vi "Custom gRPC Service Core.vi"(6 "Event Registration Refnum in":refnum<event-registration>, 11 "Node In":refnum<class "BLS Cycler Template.lvclass">) -> (2 "Server Stop":bool, 3 "Node out":refnum<class "BLS Cycler Template.lvclass">, 4 "Event Registration Refnum out":refnum<event-registration>)   [LabVIEW 2023, in "BLS Cycler Template.lvlib" / "BLS Cycler Template.lvclass"]
uses:
  BLS Cycler Template.lvclass
  C:/Program Files/National Instruments/LabVIEW 2023/vi.lib/ADAS Replay HIL/Template Node/Plugin/Template Node/Template Node.lvclass
  Custom gRPC/BLSCyclerTemplateService_server/RPC Service/BLSCyclerTemplateService/typeDefs/Server gRPC UEs.ctl
  <vilib>/gRPC/LabVIEW gRPC Library/Server API/typeDefs/gRPCId Cluster.ctl
  <vilib>/gRPC/LabVIEW gRPC Library/Shared/grpcId.ctl
  Custom gRPC/BLSCyclerTemplateService_server/RPC Messages/adas_Status.ctl
  <vilib>/ADAS Replay HIL/Template Node/Plugin/Template Node/Template Node.lvclass/Template Node.ctl
  <vilib>/ADAS Replay HIL/ADAS Plugin Utilities/AdasLvTemplate/AdasLvTemplate.lvclass/AdasLvTemplate.ctl
  <vilib>/ADAS Replay HIL/ADAS Plugin Utilities/AdasLvTemplate/AdasLvTemplate.lvclass
  <vilib>/ADAS Replay HIL/Template Node/Plugin/Template Node/Template Node.lvclass
  Custom gRPC/BLSCyclerTemplateService_server/BLSCyclerTemplateService_server.lvlib
  Custom gRPC/BLSCyclerTemplateService_server/RPC Service/BLSCyclerTemplateService/BLSCyclerTemplateService.lvclass
  <vilib>/gRPC/LabVIEW gRPC Library/grpc-lvsupport-release.lvlib
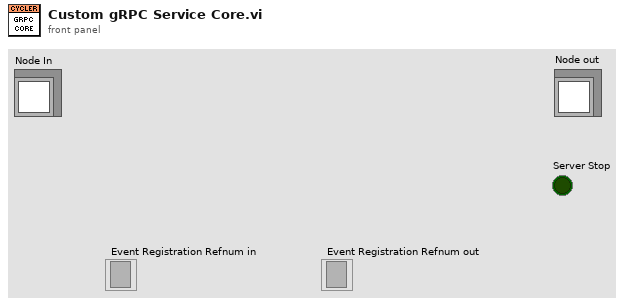
[diagram p1: front panel]
types:
  T1 = typedef "BLSCyclerTemplateService_server.lvlib/adas_Status.ctl" = cluster{"Code":i32, "Message":string}
  T2 = typedef "grpc-lvsupport-release.lvlib/grpcId.ctl" = u64
  T3 = typedef "BLSCyclerTemplateService_server.lvlib/adas_SetNumberRequest.ctl" = cluster{"SetNumber":u32}
  T4 = typedef "CIPC_buffer.lvlib/Buffer Reference.ctl" = cluster{"cipc_buffer_ref":u64, "info":T5, "settings":cluster{"prepend_array_size":bool}}
  T5 = typedef "CIPC_buffer.lvlib/Info.ctl" = cluster{"name":string, "description":string, "size":T6, "encoder":cluster{"name":string, "version":u32, "data":string}}
  T6 = typedef "CIPC_buffer.lvlib/Info Size.ctl" = cluster{"el_size_max":u32, "nr_elements":u32, "nr_elements_in_memory":u32, "frame_size":u32, "order_of_frame_size":u32, "buffer_size":u32, "order_of_buffer_size":u32}
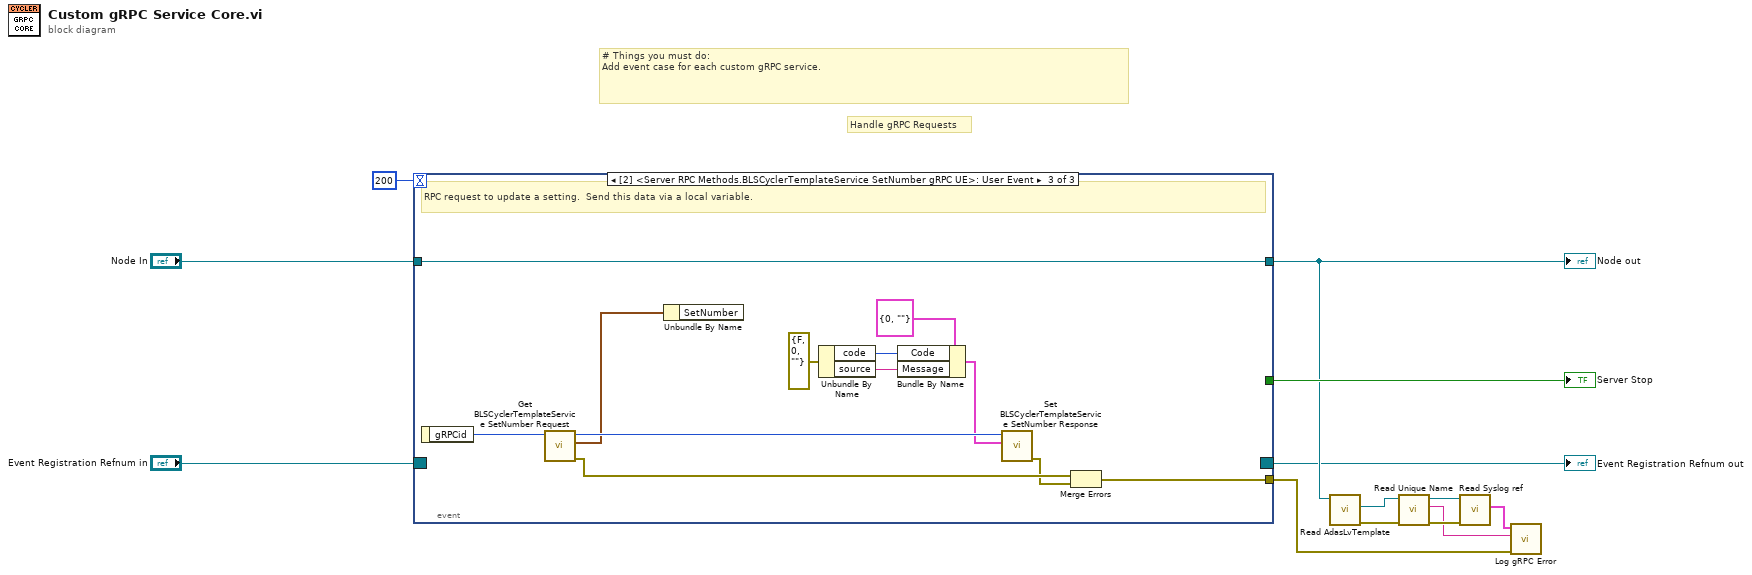
[diagram p0: block diagram]
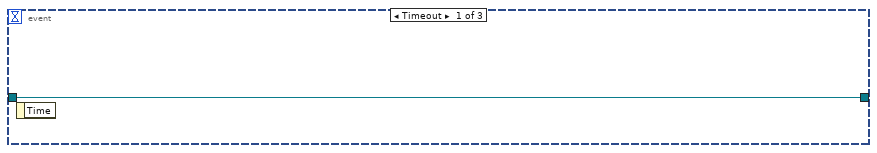
[diagram p2: hidden frame]
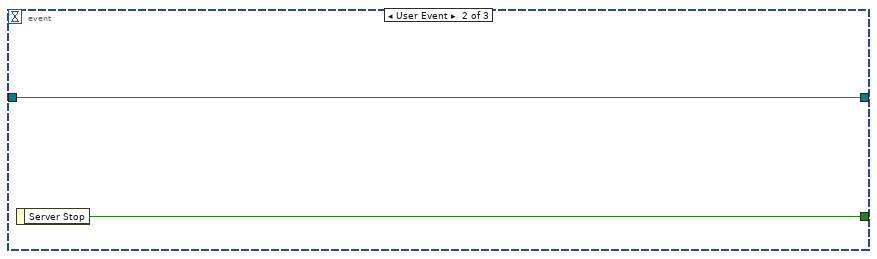
[diagram p3: hidden frame]
diagram:
  # "# Things you must do:\nAdd event case for each custom gRPC service."
  # "Handle gRPC Requests"
  n1 = event "RPC Methods Event Structure" shown="[2] <Server RPC Methods.BLSCyclerTemplateService SetNumber gRPC UE>: User Event" {
    selector: "Event Registration Refnum in" -> [_ _ _]
    dyn-events: [_ _ _] -> w1
    timeout: 200 -> [_ _ _]
    tunnel: [_ w16 _] -> w12
    tunnel: [_ _ w23] -> w4
    tunnel: "Node In" -> [w14 w15 w22]
    tunnel: [w14 w15 w22] -> w3
    event Timeout {
      n2 = event-data() -> ()  [unwired: 1 in, 1 out]
    }
    event User Event {
      n3 = event-data() -> ("Server Stop"=w16:bool)  [unwired: 1 in]
    }
    event User Event {
      # "RPC request to update a setting.  Send this data via a local variable."
      n4 = event-data() -> ("gRPCid"=w28:T2)  [unwired: 1 in]
      n5 = call "Get BLSCyclerTemplateService SetNumber Request.vi"("gRPCid in"=w28) -> ("error out"=w25:errorcluster, "Message Data"=w26:T3, "gRPCid out"=w27:T2)  [unwired: 8 in]
      n6 = Unbundle By Name(w26) -> ()  [unwired: 1 out]
      n7 = Unbundle By Name(errorcluster {"status"=FALSE, "code"=0, "source"=""} ("input cluster")) -> ("code"=w20:i32, "source"=w19:string)
      n8 = Bundle By Name(cluster=T1 {"Code"=0, "Message"=""} ("Message Data"), "Code"=w20, "Message"=w19) -> (w18:T1)
      n9 = call "Set BLSCyclerTemplateService SetNumber Response.vi"("Message Data"=w18, "gRPCid in"=w27) -> ("error out"=w24:errorcluster)  [unwired: 9 in]
      n10 = Merge Errors(w25, w24) -> (w23:errorcluster)
    }
  }
  "Server Stop" <- w12
  "Node out" <- w3
  "Event Registration Refnum out" <- w1
  n11 = call <vilib>:"Read AdasLvTemplate.vi"("Template Node in"=w3) -> ("error out"=w10:errorcluster, "AdasLvTemplate.lvlib:AdasLvTemplate.lvclass"=w11:refnum<class "AdasLvTemplate.lvclass">)  [unwired: 8 in, 1 out]
  n12 = call <vilib>:"Read Unique Name.vi"("error in"=w10, "AdasLvTemplate in"=w11) -> ("error out"=w9:errorcluster, "Unique Name"=w6:string, "AdasLvTemplate out"=w8:refnum<class "AdasLvTemplate.lvclass">)  [unwired: 7 in]
  n13 = call-dynamic "Read Syslog ref.vi"("error in (no error)"=w9, "AdasLvTemplate in"=w8) -> ("SysLog Ref"=w7:T4)  [unwired: 7 in, 2 out]
  n14 = call <vilib>:"Log gRPC Error.vi"("error in (no error)"=w4, "Plugin Unique Name"=w6, "Syslog ref in"=w7) -> ()  [unwired: 8 in, 1 out]
